vi "ClearBuffers.vi"(9 "disp size":dbl, 10 "mvc size":dbl, 11 "Num Channels":dbl) -> (1 "Disp Data":cluster{"queue out":refnum<queue>, dbl, dbl}[](array[cluster]), 2 "MVC Data":cluster{"queue out":refnum<queue>, dbl, dbl}[](array[cluster]))   [LabVIEW 2016]
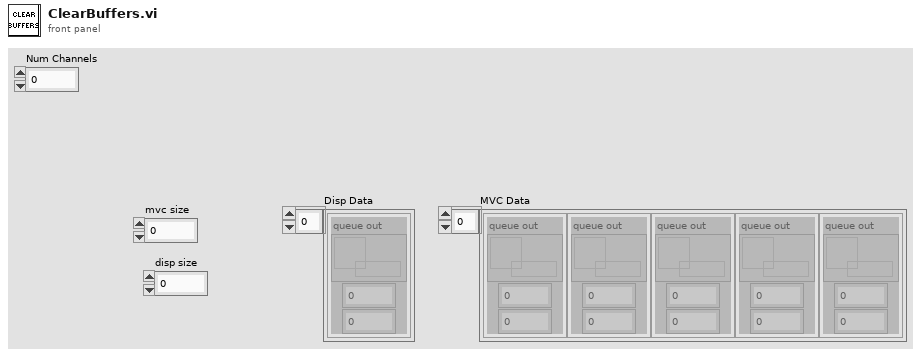
[diagram p1: front panel]
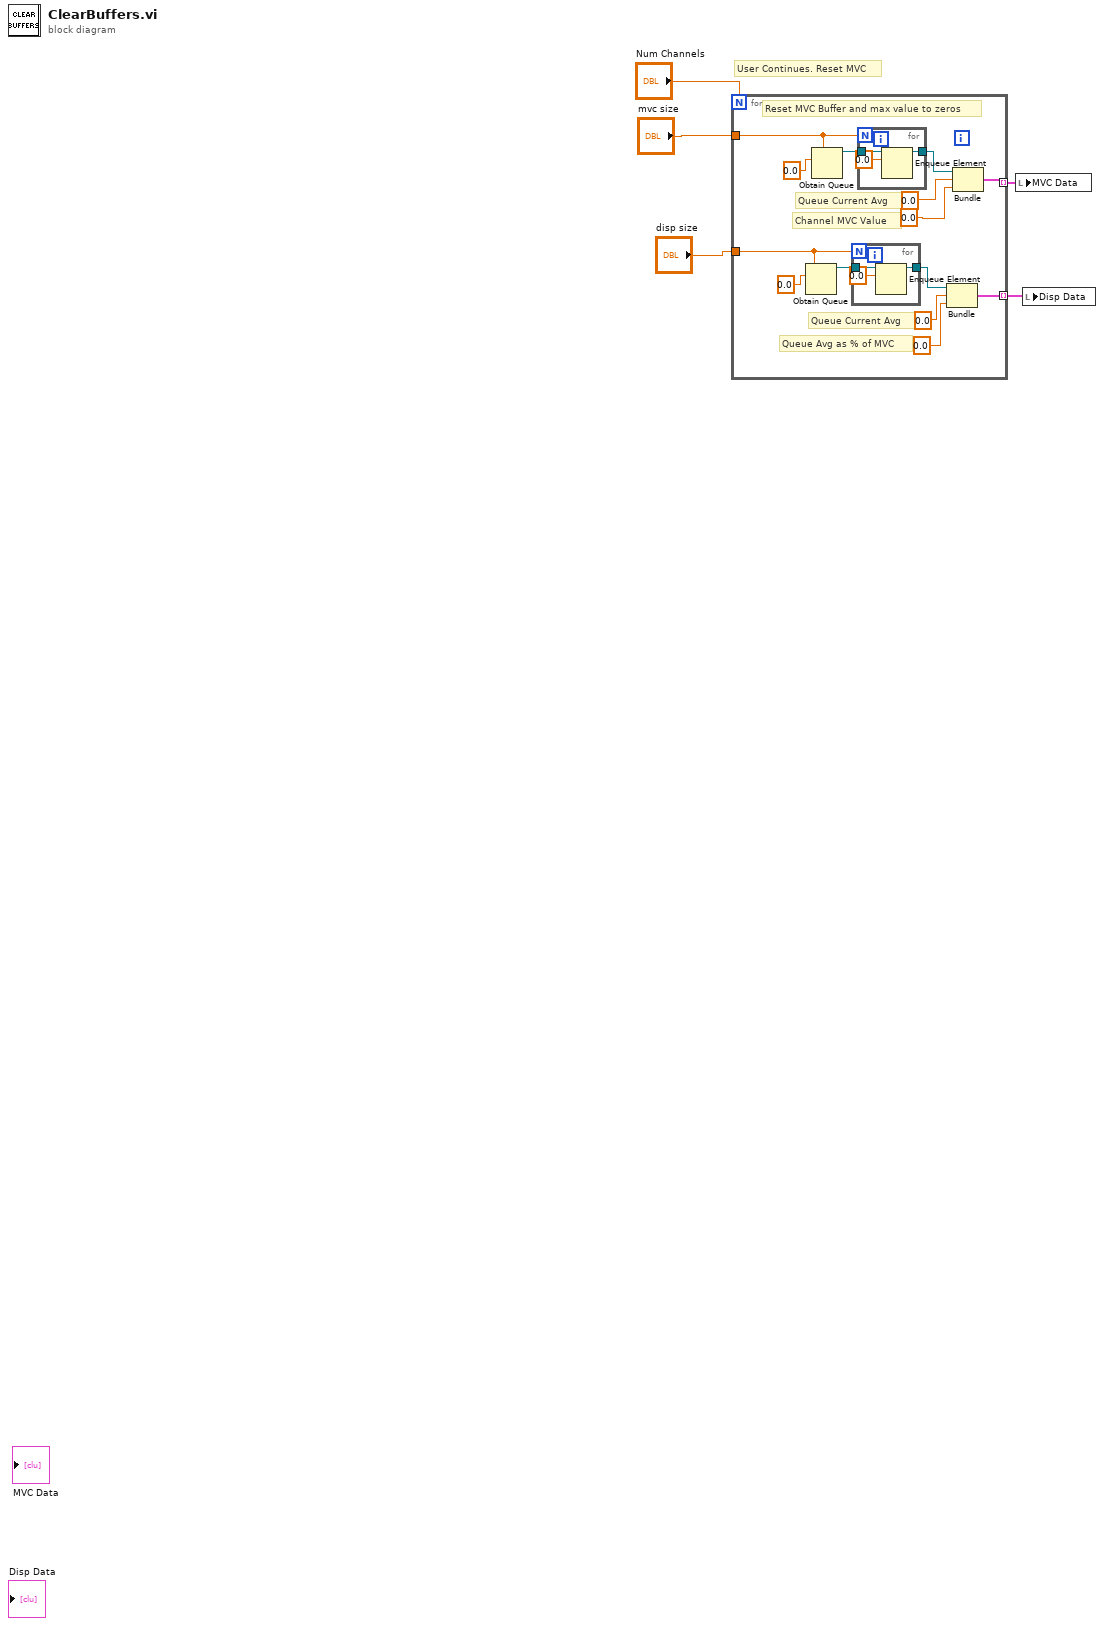
[diagram p0: block diagram]
diagram:
  # "User Continues. Reset MVC"
  n1 = for {
    N: "Num Channels" -> [_]
    tunnel: [w14] -> w5 mode=indexing
    tunnel: [w8] -> w4 mode=indexing
    tunnel: "disp size" -> [w7]
    tunnel: "mvc size" -> [w6]
    # "Queue Avg as % of MVC"
    # "Queue Current Avg"
    # "Channel MVC Value"
    # "Queue Current Avg"
    # "Reset MVC Buffer and max value to zeros"
    n2 = Obtain Queue(max queue size (-1, unlimited)=w7, element data type=0.0) -> (queue out=w9:refnum<queue>)  [unwired: 3 in, 2 out]
    n3 = Obtain Queue(max queue size (-1, unlimited)=w6, element data type=0.0) -> (queue out=w16:refnum<queue>)  [unwired: 3 in, 2 out]
    n4 = for {
      N: w7 -> [_]
      tunnel: w9 -> [w22]
      tunnel: [w20] -> w10
      n5 = Enqueue Element(queue=w22, element=0.0) -> (queue out=w20:refnum<queue>)  [unwired: 2 in, 2 out]
    }
    n6 = for {
      N: w6 -> [_]
      tunnel: w16 -> [w25]
      tunnel: [w23] -> w17
      n7 = Enqueue Element(queue=w25, element=0.0) -> (queue out=w23:refnum<queue>)  [unwired: 2 in, 2 out]
    }
    n8 = Bundle("queue out"=w10, 0.0, 0.0) -> (w8:cluster{"queue out":refnum<queue>, dbl, dbl})  [unwired: 1 in]
    n9 = Bundle("queue out"=w17, 0.0, 0.0) -> (w14:cluster{"queue out":refnum<queue>, dbl, dbl})  [unwired: 1 in]
  }
  n10 = local write "MVC Data"(w5) -> ()
  n11 = local write "Disp Data"(w4) -> ()
